vi "Point Contact Model.vi"() -> ()   [LabVIEW 2021, in "Point Contact Model.lvclass"]
uses:
  dIdV State/Point Contact Model.lvclass
  Controls/PCS Config.ctl
  Parameters.ctl
  dIdV State/Point Contact Model.lvclass/Point Contact Model.ctl
  <vilib>/Utility/config.llb/NI_LVConfig.lvlib
  <vilib>/Utility/TDMS File Viewer/NI_TDMS File Viewer.lvlib
panel:
  in  "Array - String":string[](array[string])
  in  "Input onfiguration":T1={"File Path"=path "U:/My Documents/Projects/Eremets/NV/IV/Data/August_2022/080922/m008_080922.tdms", "from scan..."=0, "...to scan"=4, "Resistance in series"=25.65079365079365, "Correct conductance "=TRUE, "Model parameters gap 1"={"Delta 1"=0.0, "Delta 2"=0.025, "Gama"=0.0, "Z"=0.0, "P"=0.0, "T"=1.0, "Integration range"=2.0, "Resolution"=0.0001}, "Scale"=1.0, "Offset"=0.0, "Other channels"=[], "Model parameters gap 2"={"Delta 1"=0.0, "Delta 2"=0.001, "Gama"=0.0, "Z"=0.0, "P"=0.0, "T"=3.8, "Integration range"=2.0, "Resolution"=0.0001}, "Gap 2 weight"=0.0, "Gnormal"=1.0} {"Gnormal" step=0.0001 format="%#_6p"; "Model parameters gap 2"."Delta 1" step=0.001 format="%#_6peV"; "Model parameters gap 2"."Resolution" format="%#_6peV"; "Model parameters gap 2"."Integration range" format="%#_6peV"; "Model parameters gap 2"."T" format="%#_6pK"; "Model parameters gap 2"."Delta 2" step=0.001 format="%#_6peV"; "Model parameters gap 2"."Gama" step=0.001 format="%#_6peV"; "Offset" scale=0.0..2.0; "Scale" scale=0.0..0.1; "Model parameters gap 1"."Delta 1" step=0.001 format="%#_6peV"; "Model parameters gap 1"."Resolution" format="%#_6peV"; "Model parameters gap 1"."Integration range" format="%#_6peV"; "Model parameters gap 1"."T" format="%#_6pK"; "Model parameters gap 1"."Delta 2" step=0.001 format="%#_6peV"; "Model parameters gap 1"."Gama" step=0.001 format="%#_6peV"; "Resistance in series" scale=0.0..80.0}
  in  "Tab Control":enum32{"Input", "Model", "Evaluations"}(tab)
  in  "View Button":bool
  out "Scans in file":i32
  out "All scans":cluster{dbl[], dbl[]}[](graph)
  in  "Open Button":bool
  out "Other values":string[](array[string])
  in  "Clear history":bool
  out "BTK model":cluster{dbl[], dbl[]}[](graph)
  out "V-I":cluster{"I":dbl[], dbl[]}[](graph)
  in  "Model Button":bool
  out "BSC Delta T":dbl=0.003040195174884819 format="%#_6peV"
  out "BSC Delta 0":dbl=0.003040195174884819 format="%#_6peV"
  in  "Physical quantities":T3={"Tc"=20.0, "T"=20.0, "Tc-> Delta factor"=1.764, "Hc2 at T"=20.0, "H"=20.0} {"H" format="%#_6pT"; "Hc2 at T" format="%#_6pT"; "Tc-> Delta factor" format="%#_6p"; "T" format="%#_6pK"; "Tc" format="%#_6pK"}
  out "BSC Delta T H":dbl=0.003040195174884819 format="%#_6peV"
  in  "Write cfg":bool
  in  "Read cfg":bool
  in  "Process Stop Button":bool
  # "<="
  # "<="
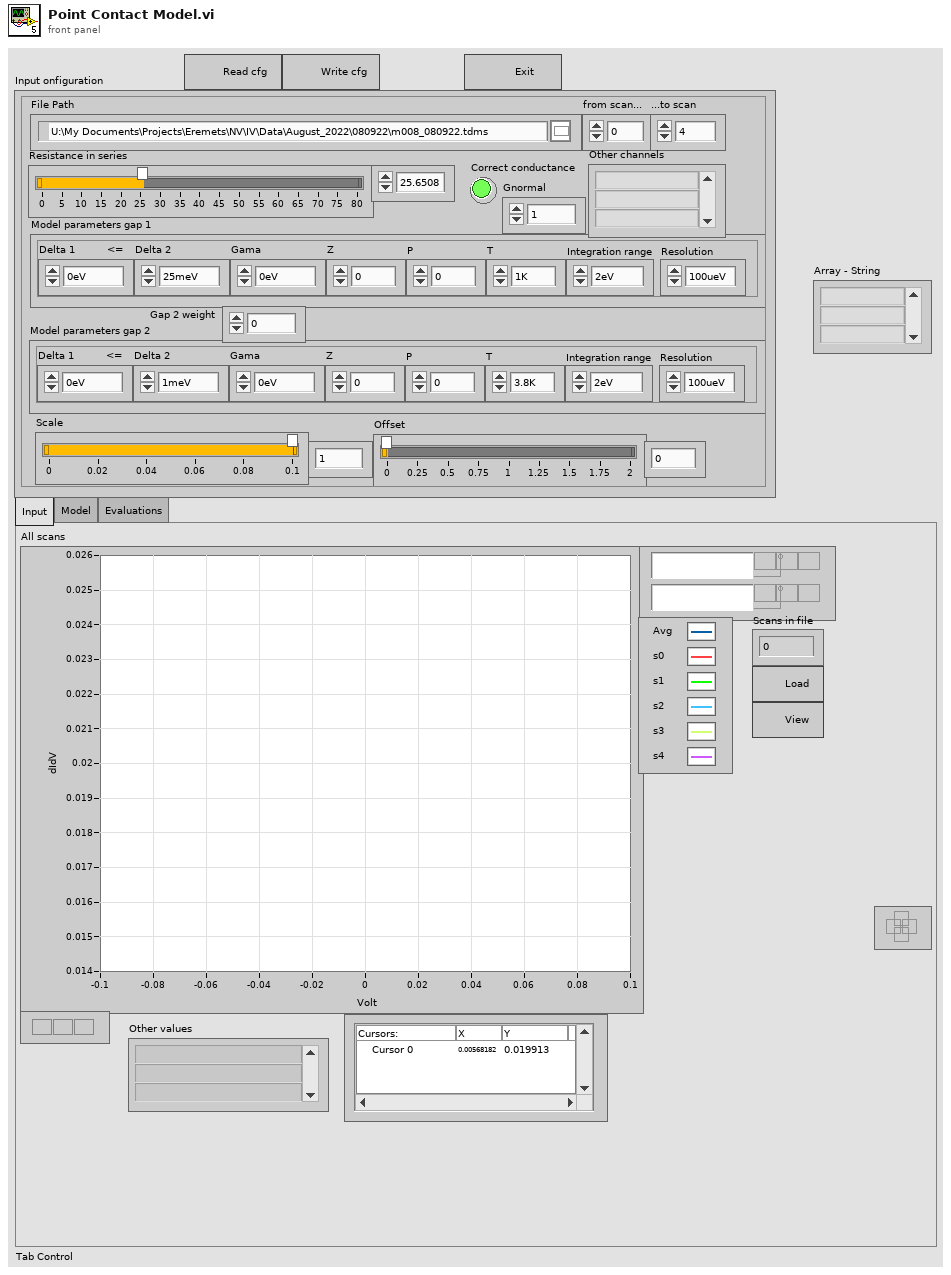
[diagram p1: front panel]
types:
  T1 = typedef "PCS Config.ctl" = cluster{"File Path":path, "from scan...":i32, "...to scan":i32, "Resistance in series":dbl, "Correct conductance ":bool, "Model parameters gap 1":T2, "Scale":dbl, "Offset":dbl, "Other channels":string[], "Model parameters gap 2":T2, "Gap 2 weight":dbl, "Gnormal":dbl}
  T2 = typedef "Parameters.ctl" = cluster{"Delta 1":dbl, "Delta 2":dbl, "Gama":dbl, "Z":dbl, "P":dbl, "T":dbl, "Integration range":dbl, "Resolution":dbl}
  T3 = cluster{"Tc":dbl, "T":dbl, "Tc-> Delta factor":dbl, "Hc2 at T":dbl, "H":dbl}
  T4 = enum8{"Enabled", "Disabled", "Disabled and Grayed Out"}
  T5 = typedef "NI_LVConfig.lvlib/Config Data RefNum.ctl" = refnum<k1>
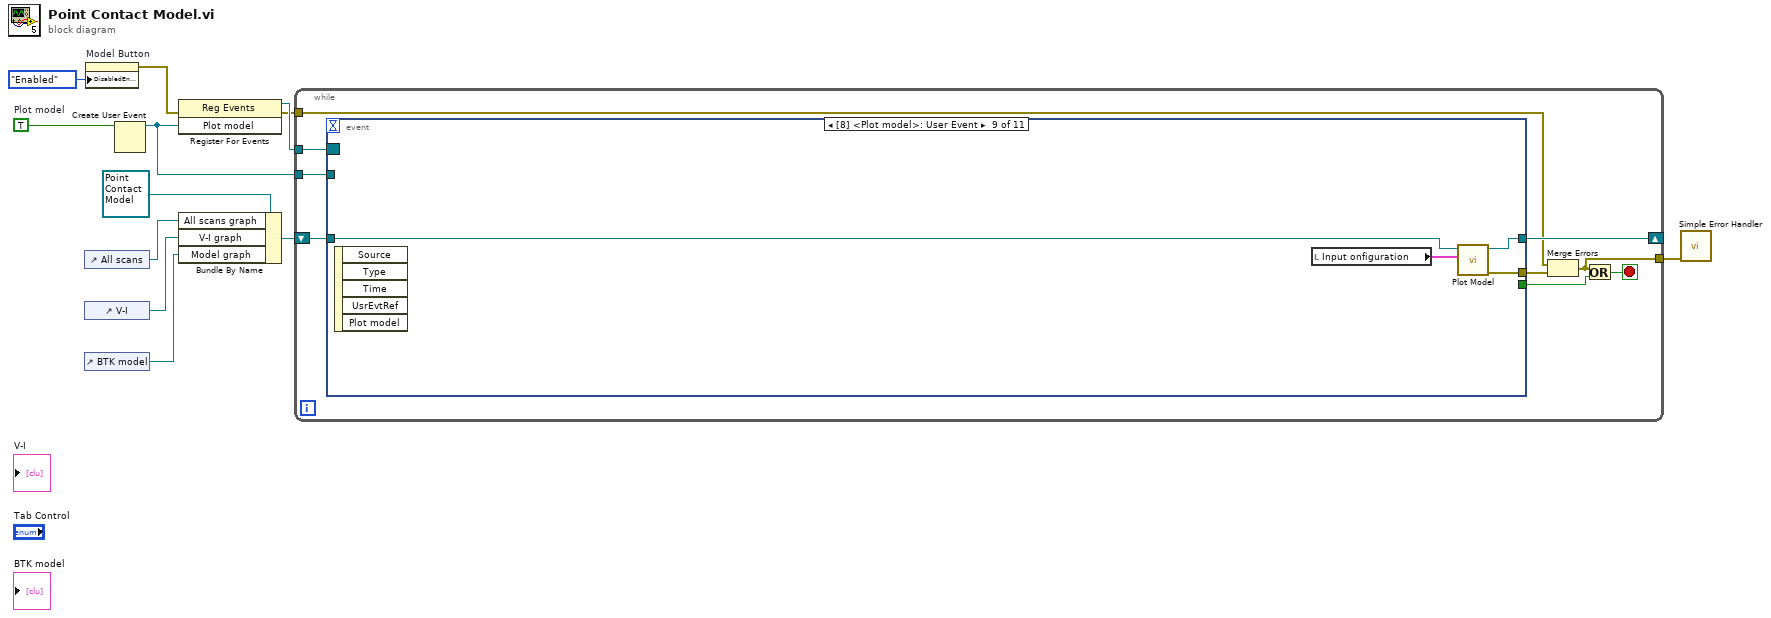
[diagram p0: block diagram]
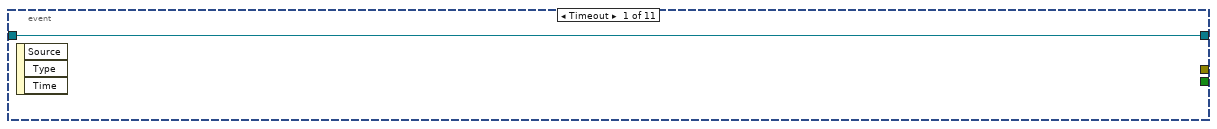
[diagram p2: hidden frame]
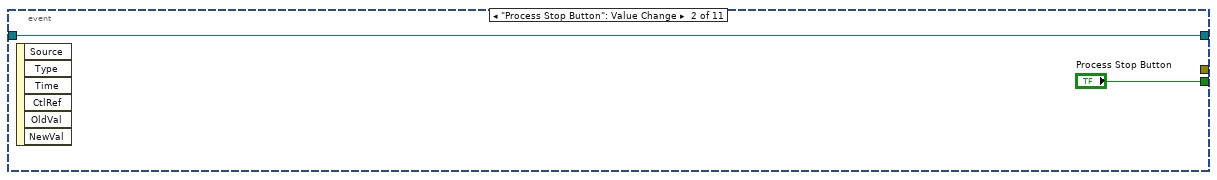
[diagram p3: hidden frame]
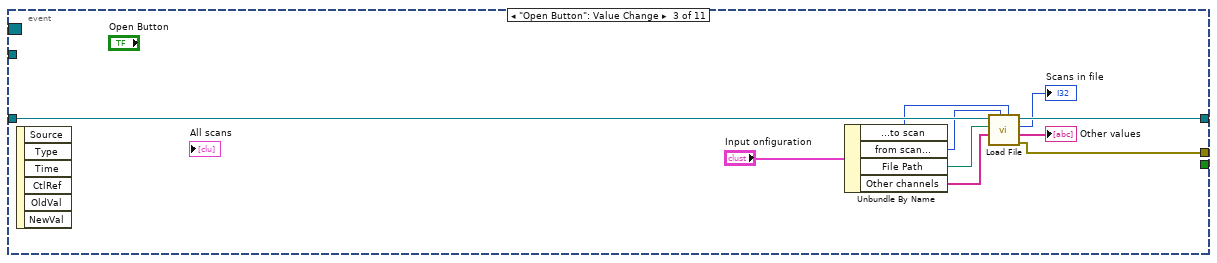
[diagram p4: hidden frame]
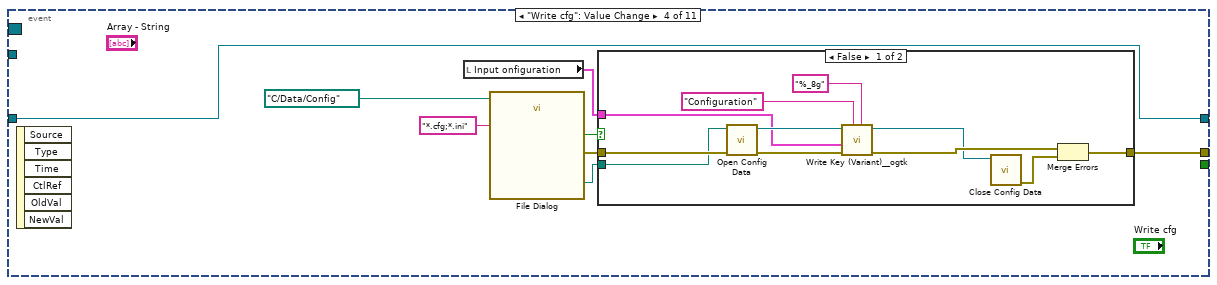
[diagram p5: hidden frame]
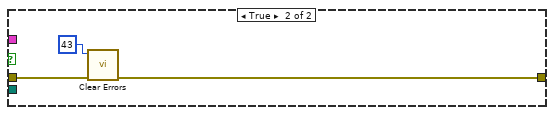
[diagram p6: hidden frame]
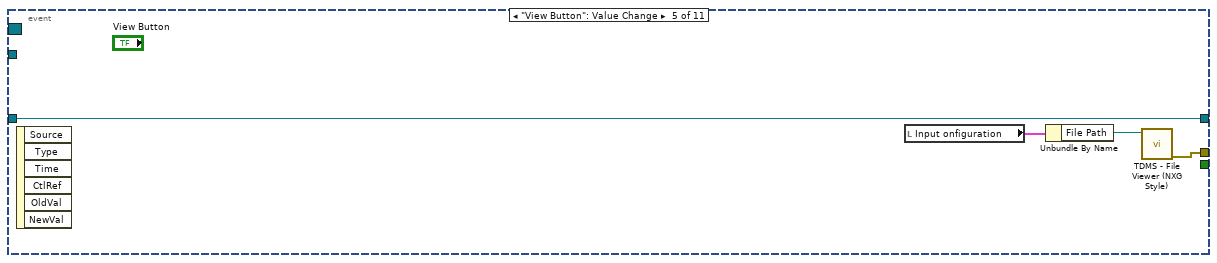
[diagram p7: hidden frame]
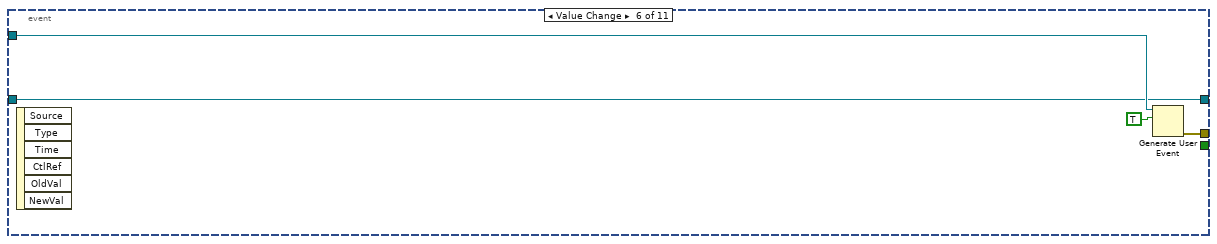
[diagram p8: hidden frame]
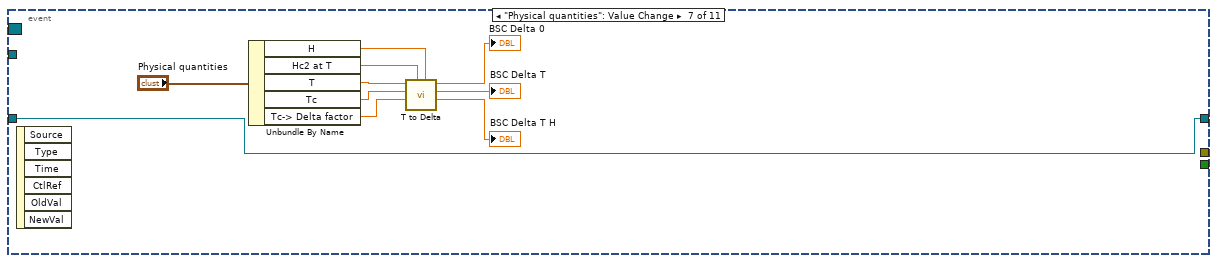
[diagram p9: hidden frame]
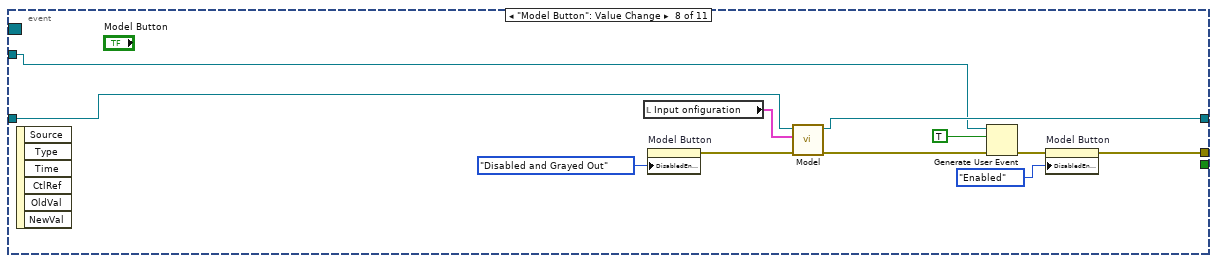
[diagram p10: hidden frame]
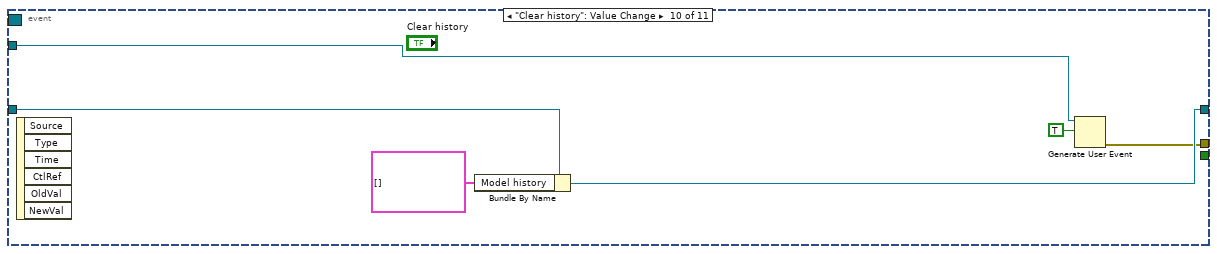
[diagram p11: hidden frame]
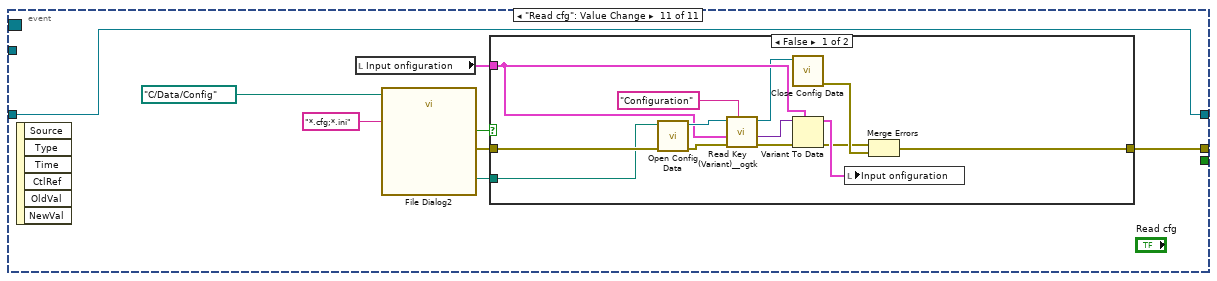
[diagram p12: hidden frame]
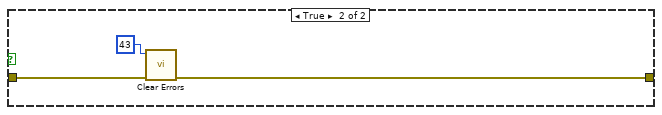
[diagram p13: hidden frame]
diagram:
  w6 = TRUE  # Plot model
  n1 = control-ref of="All scans"() -> (w10:refnum<vi>)
  n2 = control-ref of="V-I"() -> (w8:refnum<vi>)
  n3 = control-ref of="BTK model"() -> (w7:refnum<vi>)
  n4 = property on="Model Button" class="Bool"("DisabledEnum"=T4."Enabled" ("Disabled")) -> (error out=w1:errorcluster)  [unwired: 2 in, 1 out]
  n5 = Create User Event(user event datatype=w6) -> (user event=w3:refnum<user-event>)  [unwired: 1 in, 1 out]
  n6 = register-events(error in=w1, w3) -> (reference out=w5:refnum<event-registration>, error out=w4:errorcluster)  [unwired: 1 in]
  n7 = Bundle By Name(cluster=refnum<class "Point Contact Model.lvclass"> refnum ("dIdV State.lvclass"), "All scans graph"=w10, "V-I graph"=w8, "Model graph"=w7) -> (w9:refnum<class "Point Contact Model.lvclass">)
  n8 = while {
    tunnel: [w15] -> w12
    shift-right: [w17] -> _
    shift-left: w9 -> [w18]
    tunnel: w5 -> [w16]
    tunnel: w4 -> [w14]
    tunnel: w3 -> [w13]
    stop <- w20 stop-if-true
    n9 = event shown="[8] <Plot model>: User Event" {
      selector: w16 -> [_ _ _ _ _ _ _ _ _ _ _]
      dyn-events: _ -> [_ _ _ _ _ _ _ _ _ _ _]
      timeout: _ -> [_ _ _ _ _ _ _ _ _ _ _]
      tunnel: [_ "Process Stop Button" _ _ _ _ _ _ _ _ _] -> w21
      tunnel: [_ _ w32 w38 w57 w63 _ w76 w87 w91 w99] -> w19
      tunnel: w18 -> [w22 w23 w34 w37 w60 w61 w65 w85 w89 w95 w98]
      tunnel: [w22 w23 w33 w37 w60 w61 w65 w84 w88 w94 w98] -> w17
      tunnel: w13 -> [_ _ _ _ _ w64 _ w81 _ w90 _]
      event Timeout {
        n10 = event-data() -> ()  [unwired: 1 in, 3 out]
      }
      event "Process Stop Button": Value Change {
        n11 = event-data() -> ()  [unwired: 1 in, 6 out]
      }
      event "Open Button": Value Change {
        n12 = event-data() -> ()  [unwired: 1 in, 6 out]
        n13 = Unbundle By Name("Input onfiguration") -> ("...to scan"=w29:i32, "from scan..."=w28:i32, "File Path"=w27:path, "Other channels"=w25:string[])
        n14 = call-dynamic "Load File.vi"("...to scan"=w29, "from scan..."=w28, "Other channels"=w25, "File Path"=w27, "dIdV State in"=w34) -> ("error out"=w32:errorcluster, "Other values"=→"Other values":string[], "Number of scans"=→"Scans in file":i32, "dIdV State out"=w33:refnum<class "Point Contact Model.lvclass">)  [unwired: 3 in]
      }
      event "Write cfg": Value Change {
        n15 = event-data() -> ()  [unwired: 1 in, 6 out]
        n16 = local read "Input onfiguration"() -> (w36:T1)
        n17 = call "File Dialog"("start path"=path "C:/Data/Config", "pattern (all files)"="*.cfg;*.ini") -> ("selected path"=w41:path, "cancelled"=w42:bool, "error out"=w39:errorcluster)  [unwired: 10 in, 1 out]
        n18 = case shown="False" w42 {
          tunnel: w41 -> [w46 _]
          tunnel: w39 -> [w47 w56]
          tunnel: [w44 w55] -> w38
          tunnel: w36 -> [w45 _]
          frame False {
            n19 = call <vilib>:"Open Config Data.vi"("error in (no error)"=w47, "configuration file path"=w46) -> ("error out"=w49:errorcluster, "refnum"=w48:T5)  [unwired: 7 in, 1 out]
            n20 = call <userlib>:"Write Key (Variant)__ogtk.vi"("float number format"="%_8g", "section"="Configuration", "error in (no error)"=w49, "key-value"=w45, "refnum"=w48) -> ("error out"=w51:errorcluster, "refnum out"=w50:T5)  [unwired: 5 in]
            n21 = call <vilib>:"Close Config Data.vi"("refnum"=w50) -> ("error out"=w52:errorcluster)  [unwired: 9 in, 1 out]
            n22 = Merge Errors(w51, w52) -> (w44:errorcluster)
          }
          frame True {
            n23 = call <vilib>:"Clear Errors.vi"("error in (no error)"=w56, "specific error code to clear (0: all)"=43) -> ("error out"=w55:errorcluster)  [unwired: 4 in, 1 out]
          }
        }
      }
      event "View Button": Value Change {
        n24 = event-data() -> ()  [unwired: 1 in, 6 out]
        n25 = local read "Input onfiguration"() -> (w59:T1)
        n26 = Unbundle By Name(w59) -> ("File Path"=w58:path)
        n27 = call <vilib>:"TDMS - File Viewer (NXG Style).vi"("file in"=w58) -> ("error out"=w57:errorcluster)  [unwired: 9 in, 1 out]
      }
      event Value Change {
        n28 = event-data() -> ()  [unwired: 1 in, 6 out]
        n29 = Generate User Event(user event=w64, event data cluster=TRUE ("event data")) -> (error out=w63:errorcluster)  [unwired: 2 in, 1 out]
      }
      event "Physical quantities": Value Change {
        n30 = event-data() -> ()  [unwired: 1 in, 6 out]
        n31 = Unbundle By Name("Physical quantities") -> ("H"=w70:dbl, "Hc2 at T"=w69:dbl, "T"=w73:dbl, "Tc"=w72:dbl, "Tc-> Delta factor"=w71:dbl)
        n32 = call "T to Delta.vi"("H"=w70, "Hc2 at T"=w69, "Delta Tc factor"=w71, "Tc"=w72, "T"=w73) -> ("BSC Delta T H"=→"BSC Delta T H":dbl, "BSC Delta T"=→"BSC Delta T":dbl, "BSC Delta 0"=→"BSC Delta 0":dbl)  [unwired: 4 in]
      }
      event "Model Button": Value Change {
        n33 = event-data() -> ()  [unwired: 1 in, 6 out]
        n34 = local read "Input onfiguration"() -> (w83:T1)
        n35 = property on="Model Button" class="Bool"("DisabledEnum"=T4."Disabled and Grayed Out" ("Disabled")) -> (error out=w78:errorcluster)  [unwired: 2 in, 1 out]
        n36 = call-dynamic "Model.vi"("error in (no error)"=w78, "Input onfiguration"=w83, "dIdV State in"=w85) -> ("error out"=w82:errorcluster, "dIdV State out"=w84:refnum<class "Point Contact Model.lvclass">)  [unwired: 7 in]
        n37 = Generate User Event(user event=w81, event data cluster=TRUE ("event data"), error in=w82) -> (error out=w77:errorcluster)  [unwired: 1 in, 1 out]
        n38 = property on="Model Button" class="Bool"(error in=w77, "DisabledEnum"=T4."Enabled" ("Disabled")) -> (error out=w76:errorcluster)  [unwired: 1 in, 1 out]
      }
      event User Event {
        n39 = event-data() -> ()  [unwired: 1 in, 5 out]
        n40 = local read "Input onfiguration"() -> (w86:T1)
        n41 = call-dynamic "Plot Model.vi"("Input onfiguration"=w86, "dIdV State in"=w89) -> ("error out"=w87:errorcluster, "dIdV State out"=w88:refnum<class "Point Contact Model.lvclass">)  [unwired: 8 in]
      }
      event "Clear history": Value Change {
        n42 = event-data() -> ()  [unwired: 1 in, 6 out]
        n43 = Bundle By Name(cluster=w95, "Model history"=cluster{"Model V":dbl[], "Model dIdV":dbl[]}[] []) -> (w94:refnum<class "Point Contact Model.lvclass">)
        n44 = Generate User Event(user event=w90, event data cluster=TRUE ("event data")) -> (error out=w91:errorcluster)  [unwired: 2 in, 1 out]
      }
      event "Read cfg": Value Change {
        n45 = event-data() -> ()  [unwired: 1 in, 6 out]
        n46 = local read "Input onfiguration"() -> (w97:T1)
        n47 = call "File Dialog2"("start path"=path "C:/Data/Config", "pattern (all files)"="*.cfg;*.ini") -> ("selected path"=w102:path, "cancelled"=w103:bool, "error out"=w100:errorcluster)  [unwired: 10 in, 1 out]
        n48 = case shown="False" w103 {
          tunnel: w102 -> [w114 _]
          tunnel: w100 -> [w115 w119]
          tunnel: [w113 w118] -> w99
          tunnel: w97 -> [w109 _]
          frame False {
            n49 = call <vilib>:"Open Config Data.vi"("error in (no error)"=w115, "configuration file path"=w114) -> ("error out"=w106:errorcluster, "refnum"=w112:T5)  [unwired: 7 in, 1 out]
            n50 = call <userlib>:"Read Key (Variant)__ogtk.vi"("section"="Configuration", "error in (no error)"=w106, "type"=w109, "refnum"=w112) -> ("error out"=w111:errorcluster, "key-value"=w110:variant, "refnum out"=w107:T5)  [unwired: 4 in, 1 out]
            n51 = call <vilib>:"Close Config Data.vi"("refnum"=w107) -> ("error out"=w116:errorcluster)  [unwired: 9 in, 1 out]
            n52 = Variant To Data(error in=w111, type=w109, Variant=w110) -> (data=w108:T1, error out=w105:errorcluster)
            n53 = local write "Input onfiguration"(w108) -> ()
            n54 = Merge Errors(w105, w116) -> (w113:errorcluster)
          }
          frame True {
            n55 = call <vilib>:"Clear Errors.vi"("error in (no error)"=w119, "specific error code to clear (0: all)"=43) -> ("error out"=w118:errorcluster)  [unwired: 4 in, 1 out]
          }
        }
      }
    }
    n56 = Merge Errors(w14, w19) -> (w15:errorcluster)
    n57 = Or(x=w15, y=w21) -> (x .or. y?=w20:bool)
  }
  n58 = call <vilib>:"Simple Error Handler.vi"("error in (no error)"=w12) -> ()  [unwired: 4 in, 5 out]
